vi "Main.vi"() -> ()   [LabVIEW 2017, in "Acquisition.lvlib"]
doc: "This template is based off of the Queued Message Handler design pattern and the Queued Message Handler project template that ships with LabVIEW.\n\nThe main difference is that the queue is private to this module and communication between modules is performed via Broadcast and Request events.\n\nRequest events are wrapped in public API methods and are handled in the Event Handling Loop (EHL) of this VI. Any module can register for Broadcast events sent by this module. The EHL generates messages based on user interface actions.\n\nThe Message Handling Loop (MHL) processes messages generated by the EHL, or by other messages. The messages are string values, so new messages can be added easily to the Message Cases case structure in the MHL. Each message cluster can also provide an optional value for Message Data, which is a variant that can be converted to whatever message-specific data is required.\n_____\nBased on Delacor QMH Project Template 4.0.0.47.\n_____\nBased on Delacor QMH Project Template 4.1.0.56."
uses:
  Acquisition.lvlib
  <vilib>/Delacor/Delacor QMH/Libraries/Module Admin_class/Delacor_lib_QMH_Module Admin.lvclass
  Module Data--cluster.ctl
  CML Shared/Signal Type--enum.ctl
  CML Shared/Calibration Values--cluster.ctl
  Stop Argument--cluster.ctl
  <vilib>/Delacor/Delacor QMH/Libraries/Module Admin_class/Delacor_lib_QMH_Module Admin.lvclass/Delacor_lib_QMH_Module Admin.ctl
  Start Acquiring Argument--cluster.ctl
  Start Acquiring (Reply Payload)--cluster.ctl
  Stop Acquiring Argument--cluster.ctl
  Settings Editor/Update Application Settings (Reply Payload)--cluster.ctl
  Settings Editor/Settings--cluster.ctl
  <vilib>/Utility/miscctls.llb/LVPointTypeDef.ctl
  <vilib>/Delacor/Delacor QMH/Libraries/Module Admin_class/Delacor_lib_QMH_Get External Launch.vi
  <vilib>/Delacor/Delacor QMH/Libraries/Message Queue_class/Delacor_lib_QMH_Enqueue Message (Single).vi
  <vilib>/Utility/error.llb/Error Cluster From Error Code.vi
  <vilib>/ErrorRing/Error Ring.xnode
  <vilib>/Delacor/Delacor QMH/Libraries/Message Queue_class/Delacor_lib_QMH_Message Queue.lvclass
  CML Shared/CML Shared.lvlib
  Settings Editor/Settings Editor.lvlib
  Logger/Logger.lvlib
panel:
  out "Settings":T1
  out "Graph Data":waveform(dbl)[](array[waveform])
  out "error out":errorcluster
  in  "Module Admin":refnum<class "Delacor_lib_QMH_Module Admin.lvclass">
  # "This is a headless module. \nShow its panel to confirm that the Settings are updated correctly and other debugging tasks.\nUse the Settings Editor to change the settings for this module."
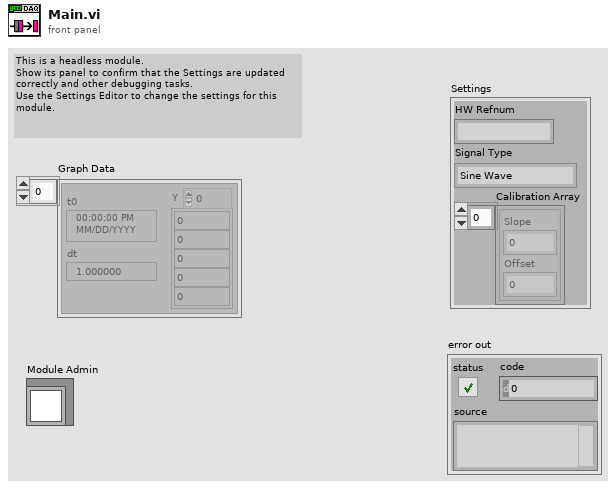
[diagram p1: front panel]
types:
  T1 = typedef "Acquisition.lvlib/Module Data--cluster.ctl" = cluster{"HW Refnum":string, "Signal Type":T2, "Calibration Array":T3[]}
  T2 = typedef "CML Shared.lvlib/Signal Type--enum.ctl" = enum16{"Sine Wave", "Square with Noise"}
  T3 = typedef "CML Shared.lvlib/Calibration Values--cluster.ctl" = cluster{"Slope":dbl, "Offset":dbl}
  T4 = typedef "Settings Editor.lvlib/Broadcast Events--cluster.ctl" = cluster{"Module Did Init":refnum<user-event>, "Status Updated":refnum<user-event>, "Error Reported":refnum<user-event>, "Module Did Stop":refnum<user-event>, "Update Module Execution Status":refnum<user-event>, "Application Settings Updated":refnum<user-event>}
  T5 = typedef "Acquisition.lvlib/Request Events--cluster.ctl" = cluster{"Stop Module":refnum<user-event>, "Show Panel":refnum<user-event>, "Hide Panel":refnum<user-event>, "Get Module Execution Status":refnum<user-event>, "Show Diagram":refnum<user-event>, "Start Acquiring":refnum<user-event>, "Stop Acquiring":refnum<user-event>, "Wakeup Helper Loop":refnum<user-event>, "Change Settings":refnum<user-event>, "Calibrate DAQ":refnum<user-event>}
  T6 = enum32{"invalid lock state", "Not Locked", "Locked (No Password)", "Password-protected"}
  T7 = typedef "Acquisition.lvlib/Stop Argument--cluster.ctl" = cluster{"Origin":string, "Exit via Stop Module Req?":bool, "Wait for Module to stop?":bool}
  T8 = typedef "Acquisition.lvlib/Start Acquiring Argument--cluster.ctl" = cluster{"Wait Notifier":refnum<notifier>}
  T9 = typedef "Acquisition.lvlib/Stop Acquiring Argument--cluster.ctl" = cluster{"Boolean":bool}
  T10 = typedef "Settings Editor.lvlib/Update Application Settings (Reply Payload)--cluster.ctl" = cluster{"Settings":T11, "Update Settings_error":errorcluster}
  T11 = typedef "Settings Editor.lvlib/Settings--cluster.ctl" = cluster{"Signal Type":T2, "Calibration Array":T3[], "Log File Base Path":path}
  T12 = typedef "LVPointTypeDef.ctl" = cluster{"Horizontal":i16, "Vertical":i16}
  T13 = enum32{"Invalid", "Standard", "Closed", "Hidden", "Minimized", "Maximized"}
  T14 = typedef "Acquisition.lvlib/Start Acquiring (Reply Payload)--cluster.ctl" = cluster{"HW ID":string, "Start Acquiring_error":errorcluster}
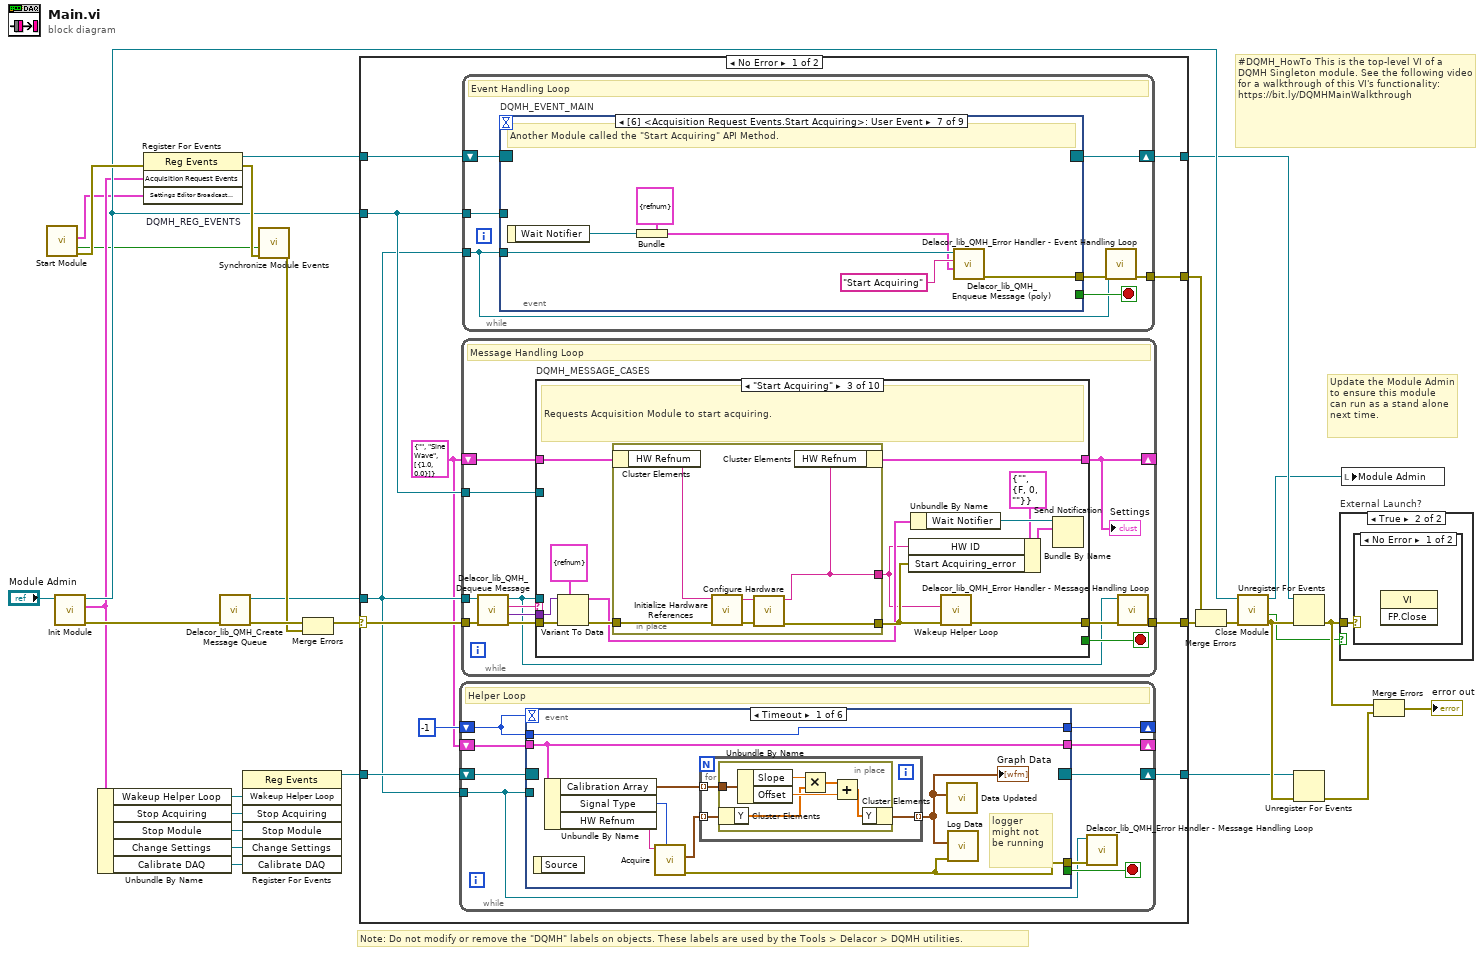
[diagram p0: block diagram]
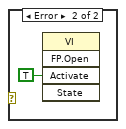
[diagram p3: hidden frame]
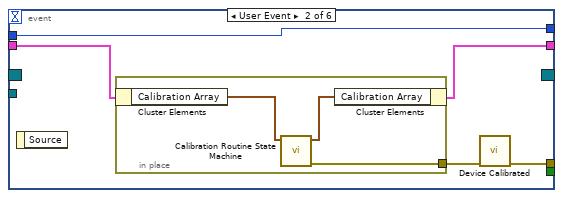
[diagram p4: hidden frame]
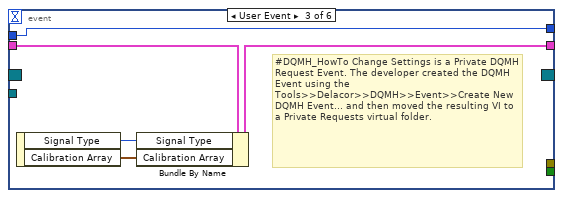
[diagram p5: hidden frame]
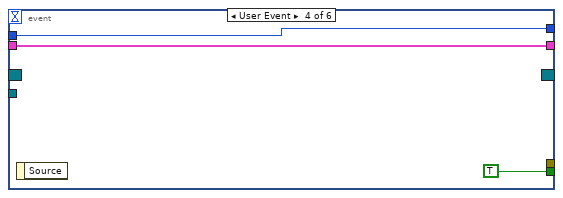
[diagram p6: hidden frame]
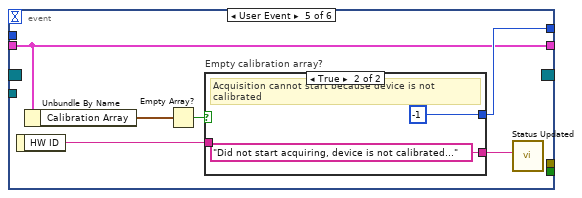
[diagram p7: hidden frame]
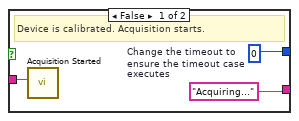
[diagram p8: hidden frame]
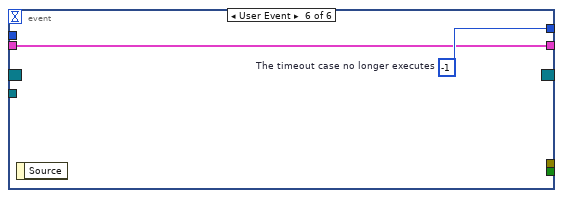
[diagram p9: hidden frame]
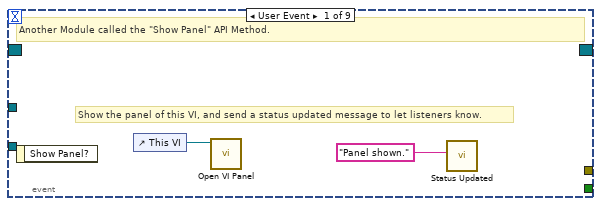
[diagram p10: hidden frame]
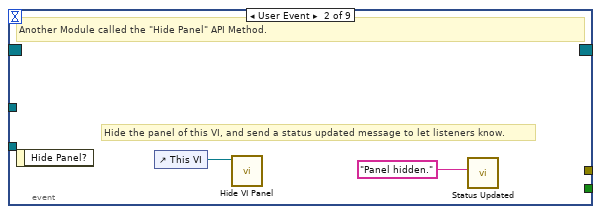
[diagram p11: hidden frame]
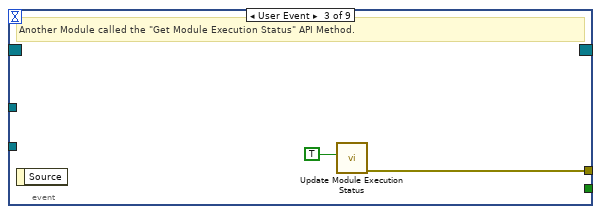
[diagram p12: hidden frame]
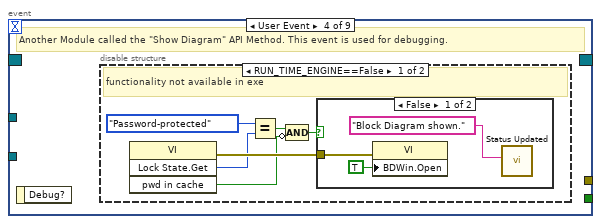
[diagram p13: hidden frame]
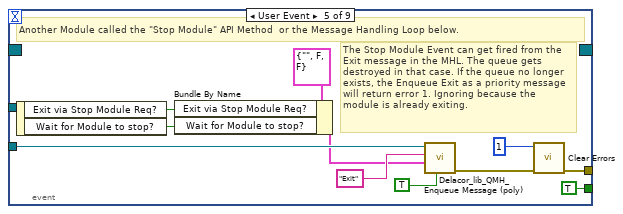
[diagram p16: hidden frame]
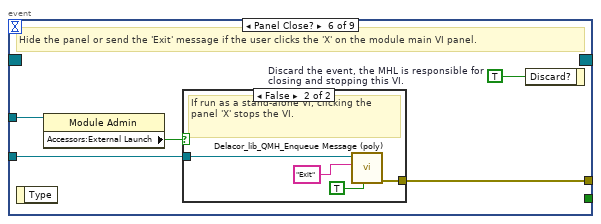
[diagram p17: hidden frame]
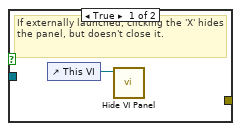
[diagram p18: hidden frame]
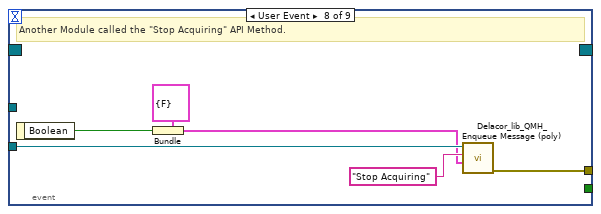
[diagram p19: hidden frame]
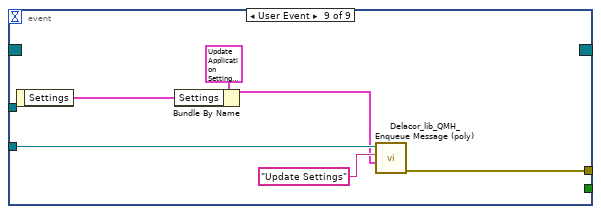
[diagram p20: hidden frame]
diagram:
  # "#DQMH_HowTo This is the top-level VI of a DQMH Singleton module. See the following video for a walkthrough of this VI's functionality: https://bit.ly/DQMHMainWalkthrough"
  # "Note: Do not modify or remove the \"DQMH\" labels on objects. These labels are used by the Tools > Delacor > DQMH utilities."
  # "Update the Module Admin to ensure this module can run as a stand alone next time."
  n1 = call "Start Module.vi"() -> ("error out"=w23:errorcluster, "Wait for Event Sync?"=w4:bool, "Settings Editor Broadcast Events"=w5:T4)  [unwired: 8 in, 1 out]
  n2 = call "Init Module.vi"("Singleton Module Admin in"="Module Admin") -> ("error out"=w29:errorcluster, "Acquisition Request Events"=w10:T5, "Singleton Module Admin out"=w17:refnum<class "Delacor_lib_QMH_Module Admin.lvclass">)  [unwired: 8 in]
  n3 = Unbundle By Name(w10) -> ("Wakeup Helper Loop"=w6:refnum<user-event>, "Stop Acquiring"=w9:refnum<user-event>, "Stop Module"=w8:refnum<user-event>, "Change Settings"=w3:refnum<user-event>, "Calibrate DAQ"=w2:refnum<user-event>)
  n4 = register-events "DQMH_REG_EVENTS"(error in=w23, w10, w5) -> (reference out=w15:refnum<event-registration>, error out=w22:errorcluster)  [unwired: 1 in]
  n5 = call <vilib>:"Delacor_lib_QMH_Create Message Queue.vi"("error in (no error)"=w29) -> ("error out"=w25:errorcluster, "Message Queue"=w14:refnum<class "Delacor_lib_QMH_Message Queue.lvclass">)  [unwired: 9 in]
  n6 = register-events(w6, w9, w8, w3, w2) -> (reference out=w7:refnum<event-registration>)  [unwired: 2 in, 1 out]
  n7 = call "Synchronize Module Events.vi"("error in (no error)"=w22, "Wait for Event Sync?"=w4) -> ("error out"=w21:errorcluster)  [unwired: 9 in]
  n8 = Merge Errors(w25, w21) -> (w24:errorcluster)
  n9 = case shown="No Error" w24 {
    selector: w24 -> [w39 w293]
    tunnel: [w41 w293] -> w30
    tunnel: [w38 w290] -> w16
    tunnel: w15 -> [w37 w290]
    tunnel: w14 -> [w33 _]
    tunnel: [w40 _] -> w28
    tunnel: w17 -> [w36 w286]
    tunnel: w7 -> [w34 w285]
    tunnel: [w31 w285] -> w1
    frame No Error {
      w32 = T1 {"HW Refnum"="", "Signal Type"=enum."Sine Wave", "Calibration Array"=[{"Slope"=1.0, "Offset"=0.0}]} ("Data Cluster")
      n10 = while {
        shift-right: [w49] -> _
        shift-left: -1 -> [w48]
        tunnel: w33 -> [w45]
        shift-right: [w44] -> _
        shift-left: w32 -> [w43]
        shift-right: [w42] -> w31
        shift-left: w34 -> [w47]
        stop <- w46 stop-if-true
        # "Helper Loop"
        n11 = event shown="[0] Timeout" {
          selector: w47 -> [_ _ _ _ _ _]
          dyn-events: [_ _ _ _ _ _] -> w42
          timeout: w48 -> [_ _ _ _ _ _]
          tunnel: [w57 w70 w80 w83 w88 w96] -> w49
          tunnel: w48 -> [w57 w70 w80 w83 _ _]
          tunnel: [_ _ _ TRUE _ _] -> w46
          tunnel: w45 -> [_ _ _ _ _ _]
          tunnel: [w58 w71 _ _ _ _] -> w50
          tunnel: [w54 w68 w78 w81 w85 w95] -> w44
          tunnel: w43 -> [w54 w69 w79 w81 w85 w95]
          event Timeout {
            # "logger\nmight not be running"
            n12 = event-data() -> ()  [unwired: 1 in, 1 out]
            n13 = Unbundle By Name(w54) -> ("Calibration Array"=w51:T3[], "Signal Type"=w56:T2, "HW Refnum"=w55:string)
            n14 = call "Acquire.vi"("Signal Type"=w56, "HW ID in"=w55) -> ("error out"=w58:errorcluster, "Graph Data"=w53:waveform(dbl)[])  [unwired: 7 in, 1 out]
            n15 = for {
              tunnel: w51 -> [w61] mode=indexing
              tunnel: w53 -> [w60] mode=indexing
              tunnel: [w59] -> w52 mode=indexing
              n16 = in-place {
                in-place-border: w61 -> [w67]
                n17 = in-place-cluster #1(w60) -> ("Y"=w62:dbl[])
                n18 = Unbundle By Name(w67) -> ("Slope"=w66:dbl, "Offset"=w64:dbl)
                n19 = Multiply(x=w66, y=w62) -> (x*y=w65:dbl[])
                n20 = Add(x=w65, y=w64) -> (x+y=w63:dbl[])
                n21 = in-place-cluster #1("Y"=w63) -> (w59:waveform(dbl))
              }
            }
            "Graph Data" <- w52
            n22 = call "Data Updated.vi"("Graph Data"=w52) -> ()  [unwired: 10 in, 1 out]
            n23 = call "Log Data.vi"("error in (no error)"=w58, "Waveforms"=w52) -> ()  [unwired: 9 in, 1 out]
          }
          event User Event {
            n24 = event-data() -> ()  [unwired: 1 in, 1 out]
            n25 = in-place {
              in-place-border: [w75] -> w72
              n26 = in-place-cluster #2(w69) -> ("Calibration Array"=w74:T3[])
              n27 = call "Calibration Routine State Machine.vi"("Calibration Array in"=w74) -> ("error out"=w75:errorcluster, "Calibration Array out"=w73:T3[])  [unwired: 9 in]
              n28 = in-place-cluster #2("Calibration Array"=w73) -> (w68:T1)
            }
            n29 = call "Device Calibrated.vi"("error in (no error)"=w72) -> ("error out"=w71:errorcluster)  [unwired: 10 in]
          }
          event User Event {
            # "#DQMH_HowTo Change Settings is a Private DQMH Request Event. The developer created the DQMH Event using the Tools>>Delacor>>DQMH>>Event>>Create New DQMH Event... and then moved the resulting VI to a Private Requests virtual folder."
            n30 = event-data() -> ("Signal Type"=w77:T2, "Calibration Array"=w76:T3[])  [unwired: 1 in]
            n31 = Bundle By Name(cluster=w79, "Signal Type"=w77, "Calibration Array"=w76) -> (w78:T1)
          }
          event User Event {
            n32 = event-data() -> ()  [unwired: 1 in, 1 out]
          }
          event User Event {
            n33 = event-data() -> ("HW ID"=w86:string)  [unwired: 1 in]
            n34 = Unbundle By Name(w85) -> ("Calibration Array"=w84:T3[])
            n35 = Empty Array?(array=w84) -> (empty?=w89:bool)
            n36 = case "Empty calibration array?" shown="True" w89 {
              tunnel: ["Acquiring..." ("Status") "Did not start acquiring, device is not calibrated..." ("Status")] -> w87
              tunnel: [w91 -1] -> w88
              tunnel: w86 -> [w92 _]
              frame False {
                w91 = 0  # Change the timeout to ensure the timeout case executes
                # "Device is calibrated. Acquisition starts."
                n37 = call "Acquisition Started.vi"("HW ID"=w92) -> ()  [unwired: 10 in, 1 out]
              }
              frame True {
                # "Acquisition cannot start because device is not calibrated"
              }
            }
            n38 = call "Status Updated.vi"("Status"=w87) -> ()  [unwired: 10 in, 1 out]
          }
          event User Event {
            w96 = -1  # The timeout case no longer executes
            n39 = event-data() -> ()  [unwired: 1 in, 1 out]
          }
        }
        n40 = call-dynamic "Delacor_lib_QMH_Error Handler - Message Handling Loop.vi"("error in (no error)"=w50, "Message Queue in"=w45) -> ()  [unwired: 8 in, 2 out]
      }
      n41 = while {
        tunnel: w33 -> [w160]
        shift-right: [w164] -> _
        shift-left: w32 -> [w165]
        tunnel: w39 -> [w168]
        tunnel: [w166] -> w41
        tunnel: w36 -> [w158]
        stop <- w163 stop-if-true
        # "Message Handling Loop"
        n42 = call-dynamic "Delacor_lib_QMH_Dequeue Message.vi"("error in (no error)"=w168, "Message Queue in"=w160) -> ("error out"=w167:errorcluster, "Message Data"=w161:variant, "Message"=w162:string, "Message Queue out"=w159:refnum<class "Delacor_lib_QMH_Message Queue.lvclass">)  [unwired: 6 in]
        n43 = case "DQMH_MESSAGE_CASES" shown="\"Start Acquiring\"" w162 {
          selector: w162 -> [_ _ _ _ _ _ _ _ _ w272]
          tunnel: w159 -> [_ _ _ _ _ _ _ w240 w263 _]
          tunnel: w167 -> [w192 w196 w209 w223 w232 w235 w237 w247 w270 w275]
          tunnel: [w189 w196 w207 w221 w231 w234 w237 w243 w267 w276] -> w169
          tunnel: w165 -> [w179 w195 w197 w218 w228 w233 w236 w242 w255 w273]
          tunnel: [w174 w195 w205 w218 w228 w233 w236 w242 w255 w273] -> w164
          tunnel: [_ _ _ _ _ _ _ _ w262 _] -> w163
          tunnel: w161 -> [_ _ w204 w220 w229 _ _ w241 w261 _]
          tunnel: w158 -> [w180 _ _ _ _ _ _ w239 w256 _]
          frame "Initialize" {
            # "Initialize - Any operation that needs to be done before the module can receive messages. Synchronize Caller Events.vi will inform Start Module.vi that the module has launched and is ready to receive messages. Module Did Init.vi will broadcast that the module initialized."
            n44 = call "Synchronize Caller Events.vi"("error in (no error)"=w192, "Singleton Module Admin in"=w180) -> ("error out"=w191:errorcluster, "Singleton Module Admin out"=w176:refnum<class "Delacor_lib_QMH_Module Admin.lvclass">)  [unwired: 8 in]
            n45 = call "Update Application Settings.vi"("wait for reply (T)"=TRUE) -> ("error out"=w188:errorcluster, "Reply Payload"=w173:T10)  [unwired: 8 in, 1 out]
            n46 = Unbundle By Name(w173) -> ("Settings.Signal Type"=w172:T2, "Settings.Calibration Array"=w171:T3[])
            n47 = property class="Module Admin"(reference=w176) -> ("Accessors:External Launch"=w184:bool)  [unwired: 1 in, 2 out]
            n48 = Bundle By Name(cluster=w179, "Signal Type"=w172, "Calibration Array"=w171) -> (w174:T1)
            n49 = Select(t=T13."Hidden" ("State"), s=w184, f=T13."Standard" ("State")) -> (s? t:f=w181:T13)
            n50 = call "Module Name--constant.vi"() -> ("Module Name"=w187:string)  [unwired: 11 in]
            n51 = property class="VI"("Front Panel.Title"=w187) -> (reference out=w186:refnum<vi>, error out=w194:errorcluster)  [unwired: 2 in]
            n52 = call "Module Name--constant.vi"() -> ("Module Name"=w177:string)  [unwired: 11 in]
            n53 = invoke class="VI" method="FP.Open"(reference=w186, error in=w194, "State"=w181) -> (reference out=w185:refnum<vi>, error out=w193:errorcluster)  [unwired: 2 in, 3 out]
            n54 = call "Module Did Init.vi"("error in (no error)"=w191, "Initialized?"=TRUE, "Origin"=w177) -> ("error out"=w190:errorcluster)  [unwired: 8 in]
            n55 = invoke class="VI" method="FP.Center"(reference=w185, error in=w193) -> ()  [unwired: 1 in, 3 out]
            n56 = Merge Errors(w190, w188) -> (w189:errorcluster)
            n57 = property on="Pane" class="Pane"("Origin"=T12 {"Horizontal"=0, "Vertical"=0}) -> ()  [unwired: 2 in, 2 out]
          }
          frame "--- Module Specific ---" {
            # "Separator -- The following cases handle messages specific to this Module."
          }
          frame "Start Acquiring" {
            # "Requests Acquisition Module to start acquiring."
            n58 = Variant To Data(error in=w209, type=T8 {"Wait Notifier"=refnum} ("Start Acquiring Argument"), Variant=w204) -> (data=w202:T8, error out=w206:errorcluster)
            n59 = in-place {
              in-place-border: [w215] -> w208
              in-place-border: w206 -> [w214]
              in-place-border: [w210] -> w198
              n60 = in-place-cluster #3(w197) -> ("HW Refnum"=w211:string)
              n61 = call "Initialize Hardware References.vi"("error in (no error)"=w214, "HW Refnum in"=w211) -> ("error out"=w213:errorcluster, "HW Refnum out"=w212:string)  [unwired: 8 in]
              n62 = call "Configure Hardware.vi"("error in (no error)"=w213, "HW Refnum in"=w212) -> ("error out"=w215:errorcluster, "HW Refnum out"=w210:string)  [unwired: 8 in]
              n63 = in-place-cluster #3("HW Refnum"=w210) -> (w205:T1)
            }
            n64 = Bundle By Name(cluster=T14 {"HW ID"="", "Start Acquiring_error"={"status"=FALSE, "code"=0, "source"=""}} ("Start Acquiring (Reply Payload)"), "HW ID"=w198, "Start Acquiring_error"=w208) -> (w200:T14)
            n65 = Unbundle By Name(w202) -> ("Wait Notifier"=w201:refnum<notifier>)
            n66 = call "Wakeup Helper Loop.vi"("error in (no error)"=w208, "HW ID"=w198) -> ("error out"=w207:errorcluster)  [unwired: 9 in]
            n67 = Send Notification(notification=w200, notifier=w201) -> ()  [unwired: 1 in, 2 out]
          }
          frame "Stop Acquiring" {
            # "Requests the Acquisition Module to stop acquiring"
            n68 = Variant To Data(error in=w223, type=T9 {"Boolean"=FALSE} ("Stop Acquiring Argument"), Variant=w220) -> (error out=w222:errorcluster)  [unwired: 1 out]
            n69 = Unbundle By Name(w218) -> ("HW Refnum"=w217:string)
            n70 = call "Stop Acquisition.vi"("error in (no error)"=w222, "HW Refnum"=w217) -> ("error out"=w221:errorcluster)  [unwired: 9 in]
            n71 = call "Acquisition Stopped.vi"("error in (no error)"=w221) -> ()  [unwired: 10 in, 1 out]
            n72 = call "Status Updated.vi"("error in (no error)"=w221, "Status"="Acquisition Stopped") -> ()  [unwired: 9 in, 1 out]
          }
          frame "Update Settings" {
            # "Send the Change Settings event to the helper loop."
            # "The Settings Editor broadcasted that the settings have changed."
            n73 = Variant To Data(error in=w232, type=T10 {"Settings"={"Signal Type"=enum."Sine Wave", "Calibration Array"=[], "Log File Base Path"=path ""}, "Update Settings_error"={"status"=FALSE, "code"=0, "source"=""}} ("Settings Updated Argument"), Variant=w229) -> (data=w226:T10, error out=w230:errorcluster)
            n74 = Unbundle By Name(w226) -> ("Settings.Signal Type"=w225:T2, "Settings.Calibration Array"=w224:T3[])
            n75 = call "Change Settings.vi"("error in (no error)"=w230, "Calibration Array"=w224, "Signal Type"=w225) -> ("error out"=w231:errorcluster)  [unwired: 8 in]
          }
          frame "---Copy This Frame---" {
            # "Duplicate this frame when creating new messages.  Change this comment in the duplicated frame to describe this message."
            n76 = Merge Errors(w235) -> (w234:errorcluster)
          }
          frame "--- Exit and Error Handling---" {
            # "Separator - The following cases handle errors and exit messages."
          }
          frame "Error" {
            # "Error - Check the error message data and respond accordingly. This message is sent by the \"Error Handler\" VIs at the end of each loop in this application."
            n77 = property class="Module Admin"(reference=w239) -> ("Accessors:External Launch"=w238:bool)  [unwired: 1 in, 2 out]
            n78 = Variant To Data(error in=w247, type=errorcluster {"status"=FALSE, "code"=0, "source"=""} ("error constant"), Variant=w241) -> (data=w248:errorcluster, error out=w245:errorcluster)
            n79 = call "Error Reported.vi"("Error"=w248) -> ()  [unwired: 10 in, 1 out]
            n80 = case shown="False" w238 {
              tunnel: [w253 _] -> w244
              tunnel: w240 -> [w251 _]
              tunnel: w248 -> [w252 _]
              frame False {
                # "If the module is running standalone, then pop up an error dialog and call the \"Exit\" message."
                n81 = call <vilib>:"Simple Error Handler.vi"("error in (no error)"=w252) -> ()  [unwired: 4 in, 5 out]
                n82 = call-poly <vilib>:"Delacor_lib_QMH_Enqueue Message (poly).vi"("Priority Message? (F)"=TRUE, "Message"="Exit", "Message Queue in"=w251) -> ("error out"=w253:errorcluster)  [unwired: 7 in, 1 out]
              }
              frame True {
                # "If the module was launched externally, calling the Error Reported broadcast VI is the only action performed by the \"Error\" message. The module's caller can then process the error appropriately."
              }
            }
            n83 = Merge Errors(w245, w244) -> (w243:errorcluster)
            n84 = local write "error out"(w243) -> ()
          }
          frame "Exit" {
            w260 = 91  # 91: not all Exit messages will have an argument
            w262 = TRUE  # Stop the VI
            # "Release the message queue reference"
            # "Exit - Exit the application."
            n85 = Variant To Data(error in=w270, type=T7 {"Origin"="", "Exit via Stop Module Req?"=FALSE, "Wait for Module to stop?"=FALSE} ("Stop Argument"), Variant=w261) -> (data=w258:T7, error out=w266:errorcluster)
            n86 = call <vilib>:"Clear Errors.vi"("error in (no error)"=w266, "specific error code to clear (0: all)"=w260) -> ("error out"=w269:errorcluster)  [unwired: 4 in, 1 out]
            n87 = Unbundle By Name(w255) -> ("HW Refnum"=w254:string)
            n88 = control-ref of="This VI"() -> (w257:refnum<vi>)
            n89 = call-dynamic "Delacor_lib_QMH_Release Message Queue.vi"("error in (no error)"=w269, "Message Queue"=w263) -> ("error out"=w268:errorcluster)  [unwired: 9 in]
            n90 = call "Handle Exit.vi"("Stop Argument"=w258, "Admin in"=w256, "VI reference"=w257) -> ("error out"=w265:errorcluster)  [unwired: 7 in, 1 out]
            n91 = call "Close Hardware References.vi"("HW Refnum in"=w254) -> ("error out"=w264:errorcluster)  [unwired: 9 in, 1 out]
            n92 = Merge Errors(w268, w265, w264) -> (w267:errorcluster)
          }
          frame Default {
            # "'Default' case only runs if there is a message that isn't defined in any of the other cases.  Output a programming error."
            n93 = call "Module Name--constant.vi"() -> ("Module Name"=w271:string)  [unwired: 11 in]
            n94 = xnode "Error Ring"("parameter 0"=w272, "parameter 1"=w271) -> ("error out"=w274:errorcluster)
            n95 = Merge Errors(w275, w274) -> (w276:errorcluster)
          }
        }
        "Settings" <- w164
        n96 = call-dynamic "Delacor_lib_QMH_Error Handler - Message Handling Loop.vi"("error in (no error)"=w169, "Message Queue in"=w159) -> ("dup error in"=w166:errorcluster)  [unwired: 8 in, 1 out]
      }
      n97 = while {
        tunnel: w33 -> [w97]
        shift-right: [w100] -> w38
        shift-left: w37 -> [w101]
        tunnel: [w102] -> w40
        tunnel: w36 -> [w98]
        stop <- w99 stop-if-true
        # "Event Handling Loop"
        n98 = event "DQMH_EVENT_MAIN" shown="[6] <Acquisition Request Events.Start Acquiring>: User Event" {
          selector: w101 -> [_ _ _ _ _ _ _ _ _]
          dyn-events: [_ _ _ _ _ _ _ _ _] -> w100
          timeout: _ -> [_ _ _ _ _ _ _ _ _]
          tunnel: [_ _ _ _ TRUE ("Discard?") _ _ _ _] -> w99
          tunnel: w97 -> [_ _ _ _ w125 w132 w144 w150 w155]
          tunnel: [_ _ w109 _ w128 w134 w145 w151 w157] -> w103
          tunnel: w98 -> [_ _ _ _ _ w131 _ _ _]
          event User Event {
            # "Show the panel of this VI, and send a status updated message to let listeners know."
            # "Another Module called the \"Show Panel\" API Method."
            n99 = event-data() -> ()  [unwired: 1 in, 1 out]
            n100 = control-ref of="This VI"() -> (w105:refnum<vi>)
            n101 = call "Open VI Panel.vi"("VI"=w105) -> ()  [unwired: 10 in, 1 out]
            n102 = call "Status Updated.vi"("Status"="Panel shown." ("format string")) -> ()  [unwired: 10 in, 1 out]
          }
          event User Event {
            # "Hide the panel of this VI, and send a status updated message to let listeners know."
            # "Another Module called the \"Hide Panel\" API Method."
            n103 = event-data() -> ()  [unwired: 1 in, 1 out]
            n104 = control-ref of="This VI"() -> (w107:refnum<vi>)
            n105 = call "Hide VI Panel.vi"("VI"=w107) -> ()  [unwired: 10 in, 1 out]
            n106 = call "Status Updated.vi"("Status"="Panel hidden." ("format string")) -> ()  [unwired: 10 in, 1 out]
          }
          event User Event {
            # "Another Module called the \"Get Module Execution Status\" API Method."
            n107 = event-data() -> ()  [unwired: 1 in, 1 out]
            n108 = call "Update Module Execution Status.vi"("Running?"=TRUE) -> ("error out"=w109:errorcluster)  [unwired: 10 in]
          }
          event User Event {
            # "Another Module called the \"Show Diagram\" API Method. This event is used for debugging."
            n109 = event-data() -> ()  [unwired: 1 in, 1 out]
            n110 = disable-structure shown="RUN_TIME_ENGINE==False" {
              frame condition #0 (active) {
                # "functionality not available in exe"
                n111 = invoke class="VI" method="Lock State.Get"() -> (error out=w115:errorcluster, "Get Lock State"=w114:T6, "pwd in cache"=w111:bool)  [unwired: 4 in, 1 out]
                n112 = Equal?(x=T6."Password-protected", y=w114) -> (x = y?=w112:bool)
                n113 = Compound Arithmetic op=AND(w112, invert w111) -> (w110:bool)
                n114 = case shown="False" w110 {
                  tunnel: w115 -> [w118 _]
                  frame False {
                    n115 = property class="VI"(error in=w118, "BDWin.Open"=TRUE ("Block Diagram Window:Open")) -> ()  [unwired: 1 in, 2 out]
                    n116 = call "Status Updated.vi"("Status"="Block Diagram shown." ("format string")) -> ()  [unwired: 10 in, 1 out]
                  }
                  frame True {
                    # "Password-protected VI, and the password is not in the cache. Do not show the diagram."
                  }
                }
              }
              frame condition #1 {
              }
            }
          }
          event User Event {
            # "The Stop Module Event can get fired from the Exit message in the MHL. The queue gets destroyed in that case. If the queue no longer exists, the Enqueue Exit as a priority message will return error 1. Ignoring because the module is already exiting."
            # "Another Module called the \"Stop Module\" API Method  or the Message Handling Loop below."
            n117 = event-data() -> ("Exit via Stop Module Req?"=w121:bool, "Wait for Module to stop?"=w120:bool)  [unwired: 1 in]
            n118 = Bundle By Name(cluster=T7 {"Origin"="", "Exit via Stop Module Req?"=FALSE, "Wait for Module to stop?"=FALSE} ("Stop Argument"), "Exit via Stop Module Req?"=w121, "Wait for Module to stop?"=w120) -> (w119:T7)
            n119 = call-poly <vilib>:"Delacor_lib_QMH_Enqueue Message (poly).vi"("Priority Message? (F)"=TRUE, "Message Data"=w119, "Message"="Exit", "Message Queue in"=w125) -> ("error out"=w129:errorcluster)  [unwired: 6 in, 1 out]
            n120 = call <vilib>:"Clear Errors.vi"("error in (no error)"=w129, "specific error code to clear (0: all)"=1) -> ("error out"=w128:errorcluster)  [unwired: 4 in, 1 out]
          }
          event Panel Close? {
            w133 = TRUE  # Discard the event, the MHL is responsible for closing and stopping this VI.
            # "Hide the panel or send the 'Exit' message if the user clicks the 'X' on the module main VI panel."
            n121 = event-data() -> ()  [unwired: 1 in, 1 out]
            n122 = property class="Module Admin"(reference=w131) -> ("Accessors:External Launch"=w130:bool)  [unwired: 1 in, 2 out]
            n123 = case shown="False" w130 {
              tunnel: w132 -> [_ w138]
              tunnel: [_ w139] -> w134
              frame True {
                # "If externally launched, clicking the 'X' hides the panel, but doesn't close it."
                n124 = control-ref of="This VI"() -> (w135:refnum<vi>)
                n125 = call "Hide VI Panel.vi"("VI"=w135) -> ()  [unwired: 10 in, 1 out]
              }
              frame False {
                # "If run as a stand-alone VI, clicking the panel 'X' stops the VI."
                n126 = call-poly <vilib>:"Delacor_lib_QMH_Enqueue Message (poly).vi"("Priority Message? (F)"=TRUE, "Message"="Exit", "Message Queue in"=w138) -> ("error out"=w139:errorcluster)  [unwired: 7 in, 1 out]
              }
            }
            n127 = event-data("Discard?"=w133) -> ()  [unwired: 1 in, 1 out]
          }
          event User Event {
            # "Another Module called the \"Start Acquiring\" API Method."
            n128 = event-data() -> ("Wait Notifier"=w140:refnum<notifier>)  [unwired: 1 in]
            n129 = Bundle(cluster=T8 {"Wait Notifier"=refnum} ("Start Acquiring Argument"), "Wait Notifier"=w140) -> (w141:T8)
            n130 = call-poly <vilib>:"Delacor_lib_QMH_Enqueue Message (poly).vi"("Message Data"=w141, "Message"="Start Acquiring", "Message Queue in"=w144) -> ("error out"=w145:errorcluster)  [unwired: 7 in, 1 out]
          }
          event User Event {
            # "Another Module called the \"Stop Acquiring\" API Method."
            n131 = event-data() -> ("Boolean"=w146:bool)  [unwired: 1 in]
            n132 = Bundle(cluster=T9 {"Boolean"=FALSE} ("Stop Acquiring Argument"), "Boolean"=w146) -> (w147:T9)
            n133 = call-poly <vilib>:"Delacor_lib_QMH_Enqueue Message (poly).vi"("Message Data"=w147, "Message"="Stop Acquiring", "Message Queue in"=w150) -> ("error out"=w151:errorcluster)  [unwired: 7 in, 1 out]
          }
          event User Event {
            n134 = event-data() -> ("Settings"=w152:T11)  [unwired: 1 in]
            n135 = Bundle By Name(cluster=T10 {"Settings"={"Signal Type"=enum."Sine Wave", "Calibration Array"=[], "Log File Base Path"=path ""}, "Update Settings_error"={"status"=FALSE, "code"=0, "source"=""}} ("Settings Updated Argument"), "Settings"=w152) -> (w154:T10)
            n136 = call-poly <vilib>:"Delacor_lib_QMH_Enqueue Message (poly).vi"("Message Data"=w154, "Message"="Update Settings", "Message Queue in"=w155) -> ("error out"=w157:errorcluster)  [unwired: 7 in, 1 out]
          }
        }
        n137 = call-dynamic "Delacor_lib_QMH_Error Handler - Event Handling Loop.vi"("error in (no error)"=w103, "Message Queue in"=w97) -> ("dup error in"=w102:errorcluster)  [unwired: 8 in, 1 out]
      }
    }
    frame Error {
      # "Synchronize Caller Events.vi will inform Start Module.vi that the module has launched and will let the code calling Start Module.vi register for broadcasts and would permit the caller receive the broadcast that an error occurred at launch time."
      n138 = call "Synchronize Caller Events.vi"("Singleton Module Admin in"=w286) -> ("error out"=w291:errorcluster)  [unwired: 9 in, 1 out]
      n139 = call "Module Name--constant.vi"() -> ("Module Name"=w289:string)  [unwired: 11 in]
      n140 = Format Into String(format string="An error occurred during initialization. %s is no longer running.", w289) -> (resulting string=w287:string)  [unwired: 2 in, 1 out]
      n141 = Merge Errors(w293, w291) -> (w292:errorcluster)
      n142 = call "Error Reported.vi"("Additional Information"=w287, "Error"=w292) -> ()  [unwired: 9 in, 1 out]
    }
  }
  n143 = Merge Errors(w28, w30) -> (w27:errorcluster)
  n144 = call "Close Module.vi"("error in (no error)"=w27, "Module Admin in"=w17) -> ("error out"=w20:errorcluster, "External Launch"=w11:bool, "Module Admin out"=w12:refnum<class "Delacor_lib_QMH_Module Admin.lvclass">)  [unwired: 7 in]
  n145 = Unregister For Events(event registration refnum=w16, error in=w20) -> (error out=w26:errorcluster)
  n146 = Unregister For Events(event registration refnum=w1, error in=w20) -> (error out=w18:errorcluster)
  n147 = case "External Launch?" shown="True" w11 {
    tunnel: w26 -> [_ w294]
    frame False {
    }
    frame True {
      n148 = case shown="No Error" w294 {
        frame No Error {
          n149 = invoke class="VI" method="FP.Close"() -> ()  [unwired: 3 in, 3 out]
        }
        frame Error {
          n150 = invoke class="VI" method="FP.Open"("Activate"=TRUE ("Activate?")) -> ()  [unwired: 4 in, 5 out]
        }
      }
    }
  }
  n151 = local write "Module Admin"(w12) -> ()
  n152 = Merge Errors(w26, w18) -> (→"error out":errorcluster)
